vi "Replace at Offset.vi"(8 "JSON to Insert":string, 9 "Offset past Item":i32, 10 "Item offset":i32, 11 "<JSON> in":string) -> (2 "Item offset":i32, 3 "<JSON>":string)   [LabVIEW 2015, in "JSONtext.lvlib"]
uses:
  JSONtext.lvlib
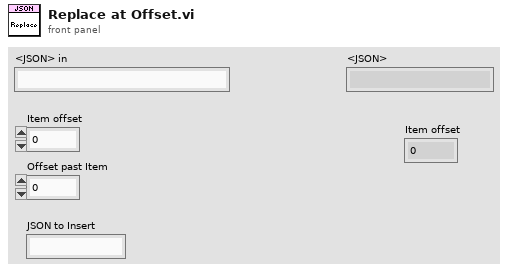
[diagram p1: front panel]
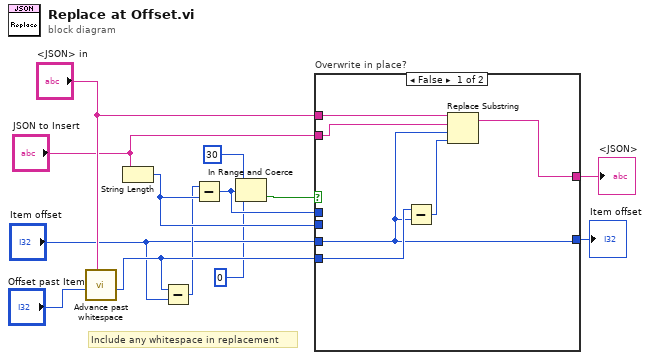
[diagram p0: block diagram]
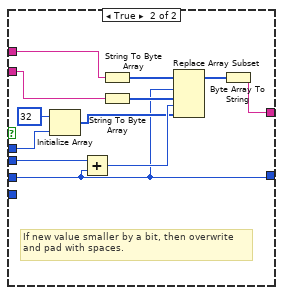
[diagram p2: hidden frame]
diagram:
  # "Include any whitespace in replacement"
  n1 = call "Advance past whitespace.vi"("JSON"="<JSON> in", "Offset"="Offset past Item") -> ("Offset of first non-whitespace"=w12:i32)  [unwired: 8 in, 1 out]
  n2 = String Length(string="JSON to Insert") -> (length=w10:i32)
  n3 = Subtract(x=w12, y="Item offset") -> (x-y=w8:i32)
  n4 = Subtract(x=w8, y=w10) -> (x-y=w9:i32)
  n5 = In Range and Coerce(upper limit=30, x=w9, lower limit=0) -> (In Range?=w6:bool)  [unwired: 1 out]
  n6 = case "Overwrite in place?" shown="False" w6 {
    tunnel: "<JSON> in" -> [w19 w28]
    tunnel: [w17 w26] -> w2
    tunnel: "JSON to Insert" -> [w18 w27]
    tunnel: "Item offset" -> [w14 w20]
    tunnel: w12 -> [w16 _]
    tunnel: w9 -> [_ w25]
    tunnel: w10 -> [_ w21]
    tunnel: [w14 w20] -> w1
    frame False {
      n7 = Subtract(x=w16, y=w14) -> (x-y=w15:i32)
      n8 = Replace Substring(2:w15, 3:w14, 4:w18, 5:w19) -> (1:w17:string)  [unwired: 1 out]
    }
    frame True {
      # "If new value smaller by a bit, then overwrite\nand pad with spaces."
      n9 = Initialize Array(u8 32, w25) -> (w23:u8[])
      n10 = Add(x=w21, y=w20) -> (x+y=w24:i32)
      n11 = String To Byte Array(string=w28) -> (unsigned byte array=w31:u8[])
      n12 = String To Byte Array(string=w27) -> (unsigned byte array=w30:u8[])
      n13 = Replace Array Subset(array=w31, new element #1=w30, index #1=w20, new element #2=w23, index #2=w24) -> (w29:u8[])
      n14 = Byte Array To String(unsigned byte array=w29) -> (string=w26:string)
    }
  }
  "<JSON>" <- w2
  "Item offset" <- w1
